vi "Write Caller Enqueuer.vi"(8 "error in (no error)":errorcluster, 10 "Actor Framework:Message Enqueuer":refnum<class "Message Enqueuer.lvclass">, 11 "Show or Hide Quick Settings Msg in":refnum<class "Show or Hide Quick Settings Msg.lvclass">) -> (0 "error out":errorcluster, 3 "Show or Hide Quick Settings Msg out":refnum<class "Show or Hide Quick Settings Msg.lvclass">)   [LabVIEW 2014, in "HIJ Vision Display.lvlib" / "Show or Hide Quick Settings Msg.lvclass"]
uses:
  Show or Hide Quick Settings Msg.lvclass
  <vilib>/ActorFramework/Message Enqueuer/Message Enqueuer.lvclass
  Show or Hide Quick Settings Msg.lvclass/Show or Hide Quick Settings Msg.ctl
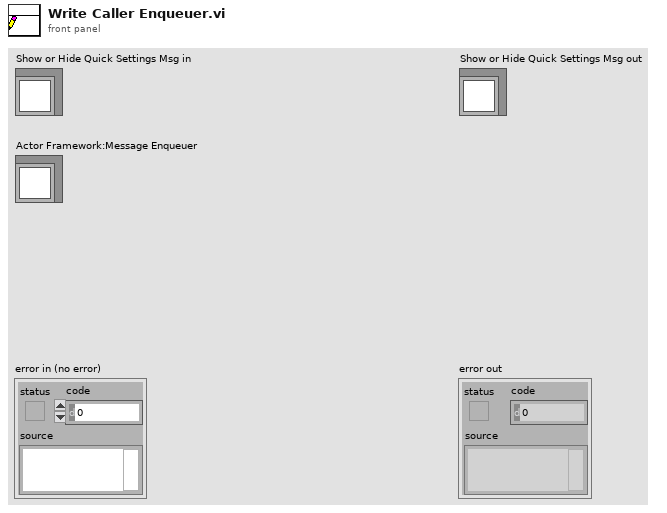
[diagram p1: front panel]
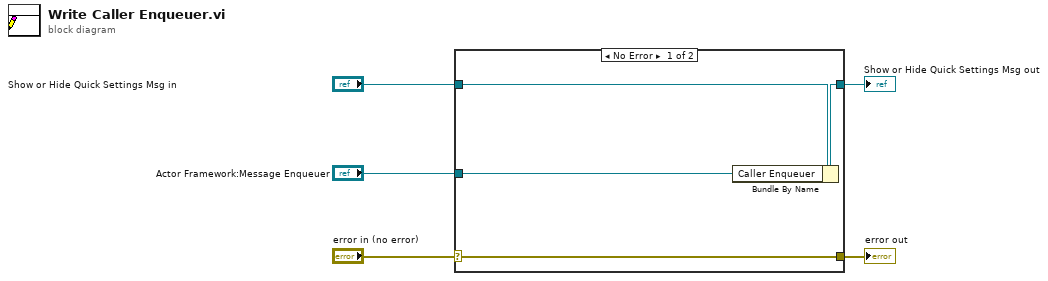
[diagram p0: block diagram]
diagram:
  n1 = case shown="No Error" "error in (no error)" {
    selector: "error in (no error)" -> [w9 w10]
    tunnel: [w9 w10] -> w4
    tunnel: [w7 w11] -> w2
    tunnel: "Show or Hide Quick Settings Msg in" -> [w8 w11]
    tunnel: "Actor Framework:Message Enqueuer" -> [w6 _]
    frame No Error {
      n2 = Bundle By Name(cluster=w8, "Caller Enqueuer"=w6) -> (w7:refnum<class "Show or Hide Quick Settings Msg.lvclass">)
    }
    frame Error {
    }
  }
  "error out" <- w4
  "Show or Hide Quick Settings Msg out" <- w2
